vi "Read Index.vi"(11 "Interlock in":refnum<class "Interlock.lvclass">) -> (2 "Index":i32=-1, 3 "Interlock out":refnum<class "Interlock.lvclass">)   [LabVIEW 2015, in "Interlocks.lvlib" / "Interlock.lvclass"]
uses:
  Interlock.lvclass
  Interlock.lvclass/Interlock.ctl
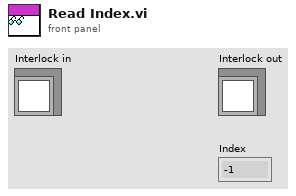
[diagram p1: front panel]
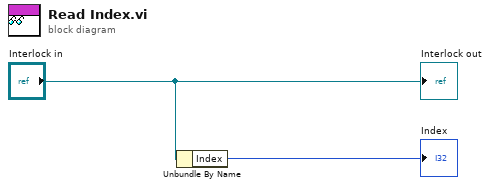
[diagram p0: block diagram]
diagram:
  n1 = Unbundle By Name("Interlock in") -> ("Index"=→"Index":i32)
  "Interlock out" <- "Interlock in"
